vi "Min_SinglePoint.vi"(8 "Error In":errorcluster, 11 "Async State Vars In":T1) -> (0 "Error Out":errorcluster, 3 "Async State Vars out":T1)   [LabVIEW 2017, in "Waveform-Processing-Custom-Device Shared.lvlib" / "Min_SP.lvlib"]
doc: "This application will provide the Minimum Set Point data"
uses:
  Min Single Point/Min_SP.lvlib
  Engine/Types/AsyncStateVariables.ctl
  <vilib>/NI VeriStand/Custom Device Waveform API/Single Waveform Read (DBL)/Single Waveform Read (DBL).lvclass
  <vilib>/NI VeriStand/Custom Device Waveform API/Single Waveform Write (DBL)/Single Waveform Write (DBL).lvclass
  <vilib>/NI Veristand/Custom Device API/Waveform Data Reference.ctl
  Engine/Types/New Async FIFOs.ctl
  <vilib>/NI/NIVS Inline Async API/_Data Access Engine/Data Access Engine/Types/Write.DVR.ctl
  <vilib>/NI/NIVS Inline Async API/_Data Access Engine/Access Type Classes/Write/Write.lvclass
  <userlib>/Circular Buffer/Controls/Circular Buffer Operations.ctl
  <vilib>/NI/NIVS Inline Async API/_Data Access Engine/Access Type Classes/Write/Write.lvclass/Write.ctl
  <vilib>/NI/NIVS Inline Async API/_Data Access Engine/Data Access Engine/Methods/Write.Data.vi
  <vilib>/NI/NIVS Inline Async API/_Data Access Engine/Access Type Classes/Write/Write.ProcessData.vi
  <userlib>/Circular Buffer/Instance VIs/Circular Buffer(2D DBL).vi
  <userlib>/Circular Buffer/Circular Buffer.lvlib
  <vilib>/NI/NIVS Inline Async API/_Data Access Engine/Data Access Engine/Data Access Engine.lvclass
  <vilib>/NI Veristand/Custom Device API/Custom Device API.lvlib
  Engine/Waveform-Processing-Custom-Device Engine.lvlib
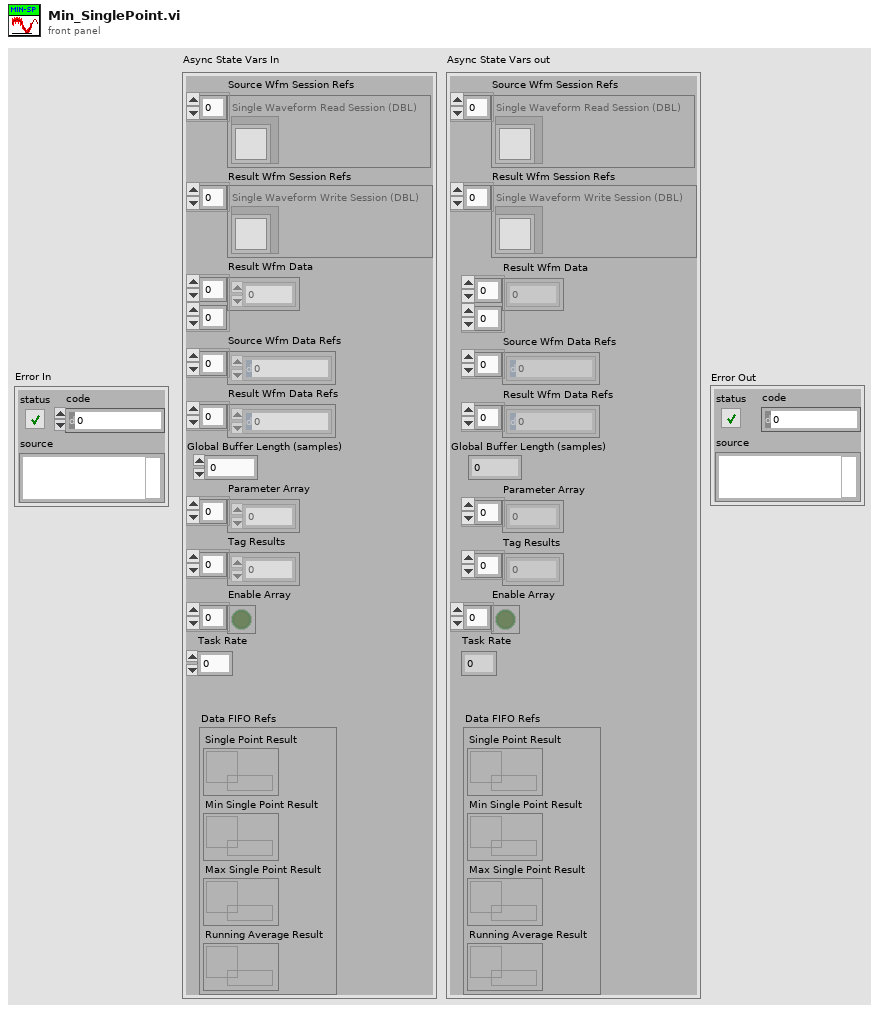
[diagram p1: front panel]
types:
  T1 = typedef "Waveform-Processing-Custom-Device Engine.lvlib/AsyncStateVariables.ctl" = cluster{"Source Wfm Session Refs":refnum<class "Single Waveform Read (DBL).lvclass">[], "Result Wfm Session Refs":refnum<class "Single Waveform Write (DBL).lvclass">[], "Result Wfm Data":dbl[][], "Source Wfm Data Refs":T2[], "Result Wfm Data Refs":T2[], "Global Buffer Length (samples)":dbl, "Parameter Array":dbl[], "Tag Results":dbl[], "Enable Array":bool[], "Task Rate":dbl, "Data FIFO Refs":T3}
  T2 = typedef "Custom Device API.lvlib/Waveform Data Reference.ctl" = i32
  T3 = typedef "Waveform-Processing-Custom-Device Engine.lvlib/New Async FIFOs.ctl" = cluster{"Single Point Result":T4, "Running Average Result":T4, "Min Single Point Result":T4, "Max Single Point Result ":T4}
  T4 = typedef "Data Access Engine.lvlib/Data Access Engine.lvclass/Write.DVR.ctl" = refnum<data-value>
  T5 = typedef "Circular Buffer.lvlib/Circular Buffer Operations.ctl" = enum16{"Initialize", "Get Backlog", "Write", "Read (continuous)", "Read (most recent)"}
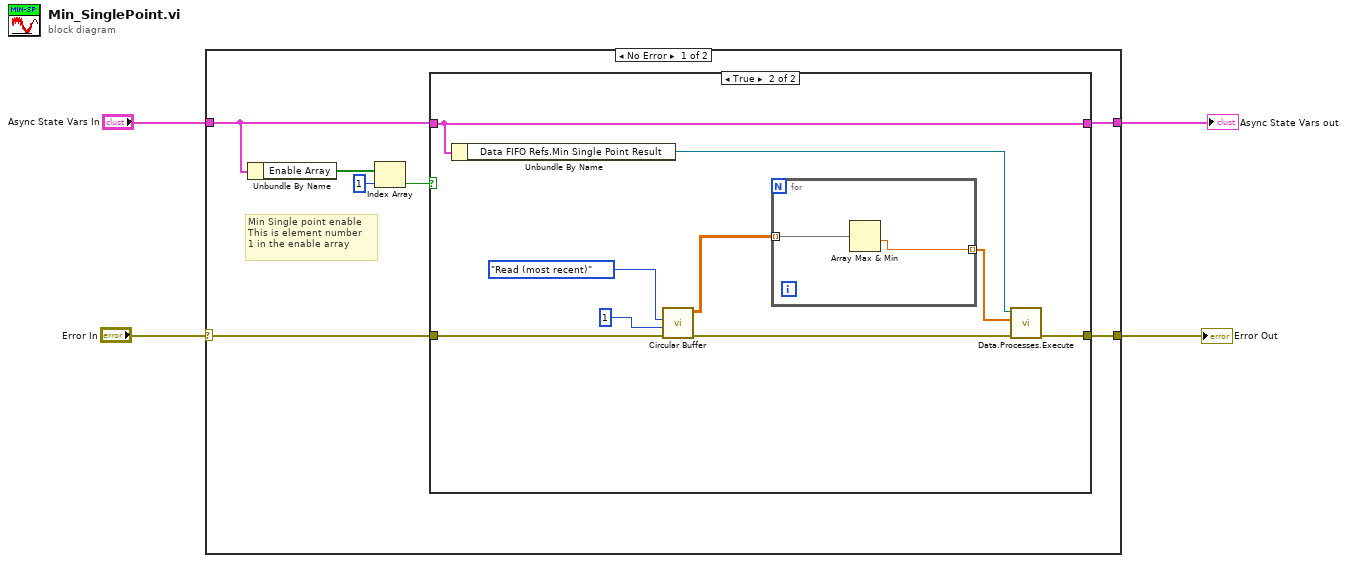
[diagram p0: block diagram]
diagram:
  n1 = case shown="No Error" "Error In" {
    selector: "Error In" -> [w11 w26]
    tunnel: [w10 w26] -> w2
    tunnel: "Async State Vars In" -> [w8 w25]
    tunnel: [w9 w25] -> w4
    frame No Error {
      # "Min Single point enable \nThis is element number\n1 in the enable array"
      n2 = Unbundle By Name(w8) -> ("Enable Array"=w7:bool[])
      n3 = Index Array(array=w7, index=1) -> (element=w5:bool)
      n4 = case shown="True" w5 {
        tunnel: w11 -> [w13 w21]
        tunnel: [w13 w17] -> w10
        tunnel: [w12 w19] -> w9
        tunnel: w8 -> [w12 w19]
        frame False {
        }
        frame True {
          n5 = Unbundle By Name(w19) -> ("Data FIFO Refs.Min Single Point Result"=w16:T4)
          n6 = call-poly <userlib>:"Circular Buffer.vi"("error in (no error)"=w21, "Read Size"=1, "Operation"=Circular_Buffer_Operations."Read (most recent)") -> ("error out"=w18:errorcluster, "Data Out"=w14:dbl[][])  [unwired: 5 in, 2 out]
          n7 = for {
            tunnel: w14 -> [w24] mode=indexing
            tunnel: [w23] -> w15 mode=indexing
            n8 = Array Max & Min(array=w24) -> (min value=w23:dbl)  [unwired: 3 out]
          }
          n9 = call-poly <vilib>:"Data.Processes.Execute.vi"("error in (no error)"=w18, "Values"=w15, "Ref"=w16) -> ("error out"=w17:errorcluster)  [unwired: 8 in]
        }
      }
    }
    frame Error {
    }
  }
  "Error Out" <- w2
  "Async State Vars out" <- w4
